vi "TopLevel.vi"(8 "error in (no error)":errorcluster) -> (0 "error out":errorcluster)   [LabVIEW 2009]
uses:
  classes/Test Suite/Test Suite.lvclass
panel:
  out "Test Report File Contents":string
  out "deleted successfully?":bool
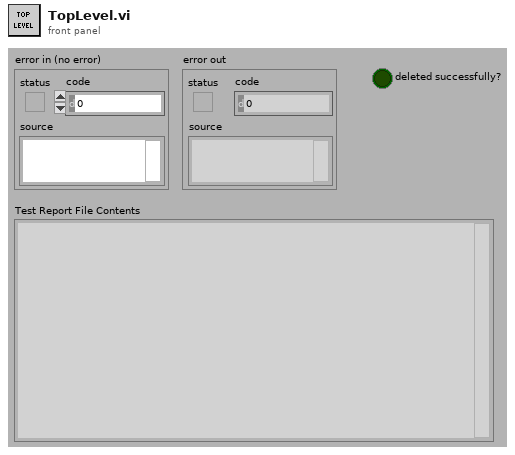
[diagram p1: front panel]
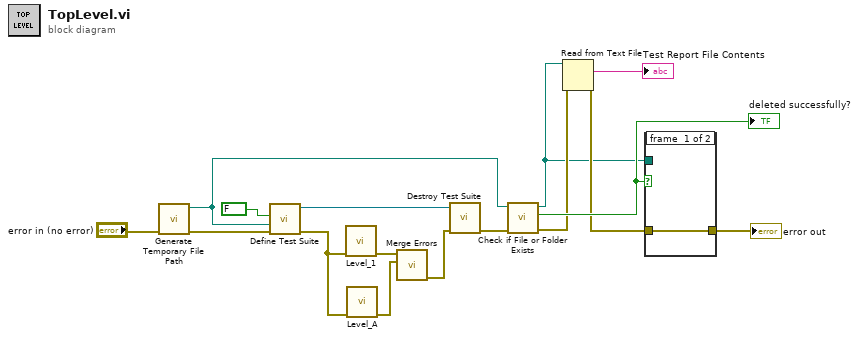
[diagram p0: block diagram]
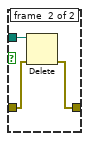
[diagram p2: hidden frame]
diagram:
  n1 = call <vilib>:"Generate Temporary File Path.vi"("error in (no error)"="error in (no error)") -> ("error out"=w12:errorcluster, "Unique Temporary File Path"=w10:path)  [unwired: 9 in]
  n2 = call "Define Test Suite.vi"("error in (no error)"=w12, "Report Path"=w10, "Interactive"=FALSE) -> ("error out"=w2:errorcluster, "Test Suite"=w14:refnum<class "Test Suite.lvclass">)  [unwired: 7 in]
  n3 = call "Level_1.vi"("error in (no error)"=w2) -> ("error out"=w16:errorcluster)  [unwired: 10 in]
  n4 = call "Level_A.vi"("error in (no error)"=w2) -> ("error out"=w15:errorcluster)  [unwired: 10 in]
  n5 = call <vilib>:"Merge Errors.vi"("error in 2 (no error)"=w15, "error in 1 (no error)"=w16) -> ("error out"=w1:errorcluster)  [unwired: 5 in]
  n6 = call-dynamic "Destroy Test Suite.vi"("error in (no error)"=w1, "Test Suite in"=w14) -> ("error out"=w11:errorcluster)  [unwired: 9 in]
  n7 = call <vilib>:"Check if File or Folder Exists.vi"("error in (no error)"=w11, "path"=w10) -> ("error out"=w8:errorcluster, "file or folder exists?"=w9:bool, "dup path"=w5:path)  [unwired: 7 in]
  "deleted successfully?" <- w9
  n8 = Read from Text File(file (use dialog)=w5, error in=w8) -> (text=→"Test Report File Contents":string, error out=w7:errorcluster)  [unwired: 2 in, 2 out]
  n9 = case shown="True" w9 {
    tunnel: w5 -> [_ w20]
    tunnel: w7 -> [w17 w19]
    tunnel: [w17 w18] -> w4
    frame #0 {
    }
    frame #1 {
      n10 = Delete(path (use dialog)=w20, error in=w19) -> (error out=w18:errorcluster)  [unwired: 3 in, 2 out]
    }
  }
  "error out" <- w4
